vi "Crop Supercell to new subcell.vi"(8 "New Lattice Vector c":dbl[](array[numeric])=[0.0, 0.0, 6.0], 9 "New Lattice Vector b":dbl[](array[numeric])=[0.0, 6.0, 0.0], 10 "New Lattice Vector a":dbl[](array[numeric])=[6.0, 0.0, 0.0], 11 "Supercell Structure":T1={"Structure Name"="CdTe Expanded to Box", "Lattice vector a"=[19.0, 0.0, 0.0], "Lattice vector b"=[0.0, 90.0, 0.0], "Lattice vector c"=[0.0, 0.0, 19.98181818181818], "Atoms Array"=[{"Atom Name"="Cd", "Positions (Direct)"=array501x3[1503 elements], "Positions (Cartesian)"=array501x3[1503 elements]}, {"Atom Name"="Te", "Positions (Direct)"=array504x3[1512 elements], "Positions (Cartesian)"=array504x3[1512 elements]}], "# of atoms"=1005} {"Atoms Array"."Positions (Cartesian)" format="%#_4g"; "Atoms Array"."Positions (Direct)" format="%#_4f"}) -> (3 "Reduced Structure":T1={"Structure Name"="Reduced CdTe Expanded to Box", "Lattice vector a"=[6.0, 0.0, 0.0], "Lattice vector b"=[0.0, 6.0, 0.0], "Lattice vector c"=[0.0, 0.0, 6.0], "Atoms Array"=[{"Atom Name"="Cd", "Positions (Direct)"=[[0.00016666666666666666, 0.00016666666666666666, 0.16881746031746028], [0.00016666666666666666, 0.04433375914924137, 0.9472432736655599], [0.00016666666666666666, 0.7785924800147661, 0.12465036783488567], [0.00016666666666666666, 0.8227595724973409, 0.9030761811829852], [0.5514821294214376, 0.41146311958200377, 0.5359468207502227]], "Positions (Cartesian)"=[[0.0, 0.0, 1.0119047619047619], [0.0, 0.2650025548954482, 5.6824596419933595], [0.0, 4.670554880088597, 0.7469022070093141], [0.0, 4.935557434984045, 5.417457087097911], [3.307892776528626, 2.4677787174920227, 3.2146809245013364]]}, {"Atom Name"="Te", "Positions (Direct)"=[[0.2758243980440521, 0.022250212907954016, 0.5580303669915101], [0.2758243980440521, 0.8006760262560535, 0.5138632745089352], [0.8271398607988233, 0.3893795733407164, 0.14673391407617298], [0.8271398607988233, 0.43354666582329104, 0.9251597274242727]], "Positions (Cartesian)"=[[1.653946388264313, 0.1325012774477241, 3.3471822019490607], [1.653946388264313, 4.803056157536321, 3.0821796470536116], [4.96183916479294, 2.3352774400442984, 0.879403484457038], [4.96183916479294, 2.6002799949397466, 5.549958364545636]]}], "# of atoms"=9} {"Atoms Array"."Positions (Cartesian)" format="%#_4f"; "Atoms Array"."Positions (Direct)" format="%#_4f"})   [LabVIEW 2010]
uses:
  <vilib>/Analysis/baseanly.llb/Real Inverse Matrix.vi
  <vilib>/Analysis/baseanly.llb/A x Vector.vi
  <vilib>/Analysis/NI_AALBase.lvlib
panel:
  out "Stoichiometry":i32[](array[numeric])=[5, 4]
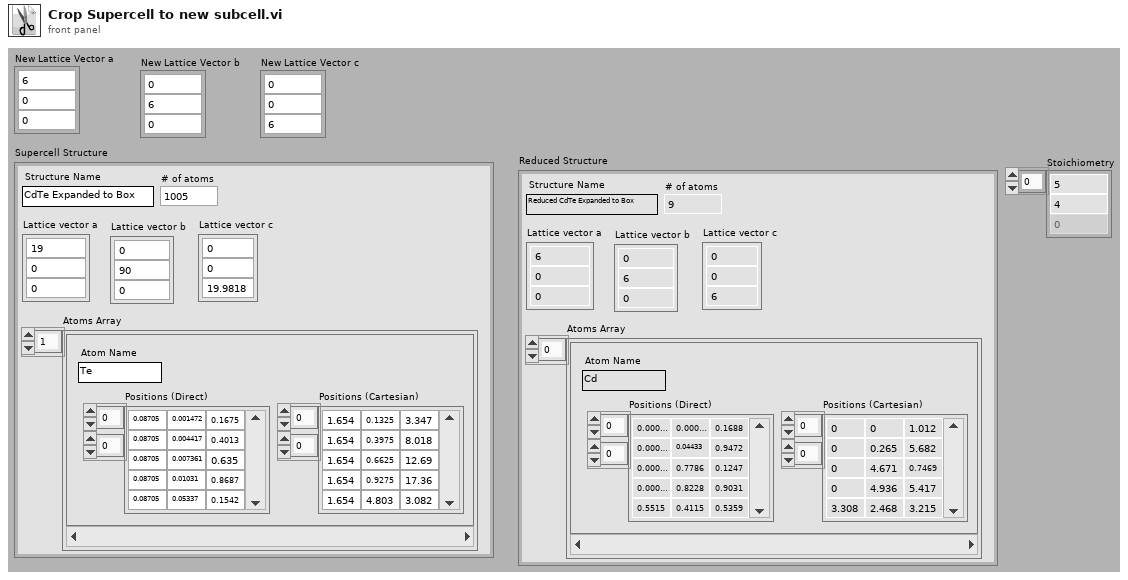
[diagram p1: front panel]
types:
  T1 = cluster{"Structure Name":string, "Lattice vector a":dbl[], "Lattice vector b":dbl[], "Lattice vector c":dbl[], "Atoms Array":cluster{"Atom Name":string, "Positions (Direct)":dbl[][], "Positions (Cartesian)":dbl[][]}[], "# of atoms":i32}
  T2 = typedef "NI_Matrix.lvlib/RealMatrix.ctl" = dbl[][]
  T3 = cluster{"Atom Name":string, "Positions (Direct)":dbl[][], "Positions (Cartesian)":dbl[][]}[]
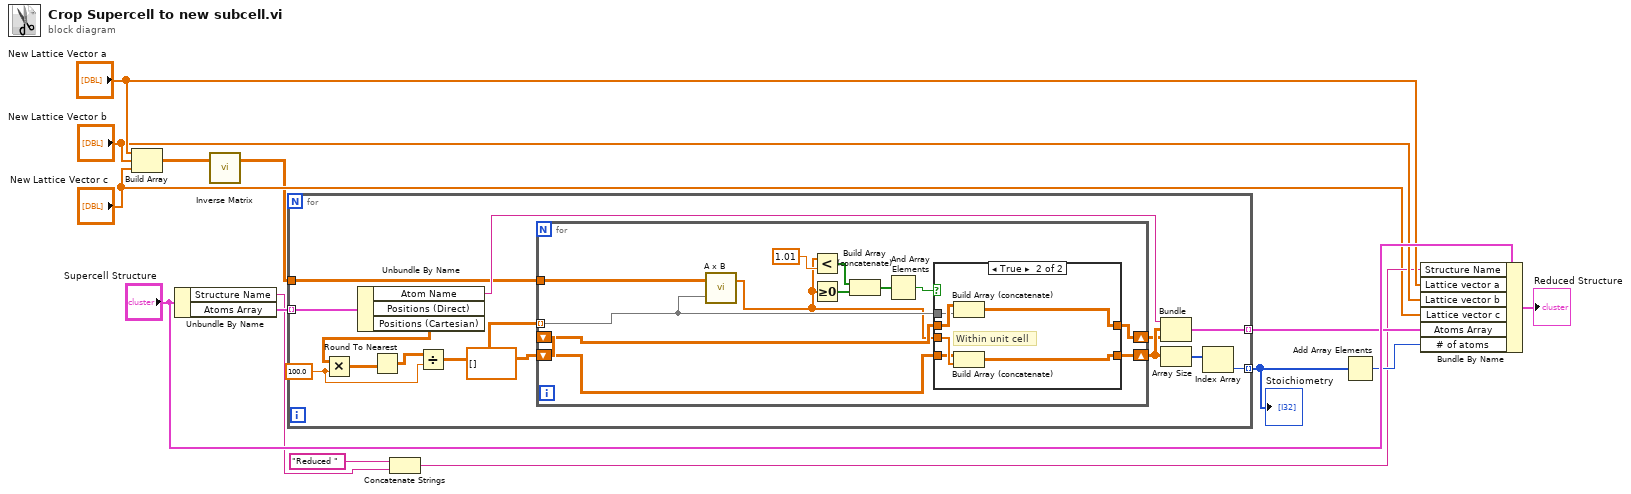
[diagram p0: block diagram]
diagram:
  n1 = Build Array("New Lattice Vector a", "New Lattice Vector b", "New Lattice Vector c") -> (w10:T2)
  n2 = Unbundle By Name("Supercell Structure") -> ("Structure Name"=w4:string, "Atoms Array"=w14:T3)
  n3 = call-poly <vilib>:"Inverse Matrix.vi"("Input Matrix"=w10) -> ("Inverse Matrix"=w1:T2)  [unwired: 1 in, 1 out]
  n4 = for {
    tunnel: w14 -> [w28] mode=indexing
    tunnel: [w26] -> w12 mode=indexing
    tunnel: w1 -> [w25]
    tunnel: [w20] -> w7 mode=indexing
    w16 = 100.0 ("y")
    w23 = dbl[][] []
    n5 = Unbundle By Name(w28) -> ("Atom Name"=w27:string, "Positions (Cartesian)"=w19:dbl[][])  [unwired: 1 out]
    n6 = Multiply(x=w19, y=w16) -> (x*y=w18:dbl[][])
    n7 = Round To Nearest(number=w18) -> (nearest integer value=w17:dbl[][])
    n8 = Divide(x=w17, y=w16) -> (x/y=w15:dbl[][])
    n9 = for {
      tunnel: w25 -> [w40]
      tunnel: w15 -> [w30] mode=indexing
      shift-right: [w39] -> w24
      shift-left: w23 -> [w38]
      shift-right: [w36] -> w22
      shift-left: w23 -> [w37]
      n10 = call-poly <vilib>:"A x B.vi"("Vector"=w30, "A"=w40) -> ("A x Vector"=w29:dbl[])  [unwired: 1 out]
      n11 = Less?(x=w29, y=1.01) -> (x < y?=w33:bool[])
      n12 = Greater Or Equal To 0?(x=w29) -> (x >= 0?=w31:bool[])
      n13 = Build Array (concatenate)(w33, w31) -> (w32:bool[])
      n14 = And Array Elements(Boolean array=w32) -> (logical AND=w34:bool)
      n15 = case shown="True" w34 {
        tunnel: w29 -> [_ w48]
        tunnel: [w42 w47] -> w39
        tunnel: w38 -> [w42 w46]
        tunnel: w30 -> [_ w44]
        tunnel: w37 -> [w41 w45]
        tunnel: [w41 w43] -> w36
        frame False {
          # "Outside the new unit cell"
        }
        frame True {
          # "Within unit cell"
          n16 = Build Array (concatenate)(w45, w44) -> (w43:dbl[][])
          n17 = Build Array (concatenate)(w46, w48) -> (w47:dbl[][])
        }
      }
    }
    n18 = Bundle("Atom Name"=w27, w24, w22) -> (w26:cluster{"Atom Name":string, dbl[][], dbl[][]})  [unwired: 1 in]
    n19 = Array Size(array=w24) -> (size(s)=w21:i32[])
    n20 = Index Array(array=w21) -> (element=w20:i32)  [unwired: 1 in]
  }
  "Stoichiometry" <- w7
  n21 = Concatenate Strings("Reduced " ("Structure Name"), w4) -> (w3:string)
  n22 = Add Array Elements(numeric array=w7) -> (sum=w6:i32)
  n23 = Bundle By Name(cluster="Supercell Structure", "Structure Name"=w3, "Lattice vector a"="New Lattice Vector a", "Lattice vector b"="New Lattice Vector b", "Lattice vector c"="New Lattice Vector c", "Atoms Array"=w12, "# of atoms"=w6) -> (→"Reduced Structure":T1)
